vi "Actor Core.vi"(8 "error in":errorcluster, 11 "Nested in":refnum<class "GUI.lvclass">) -> (0 "error out":errorcluster, 3 "Actor out":refnum<class "Actor.lvclass">)   [LabVIEW 2020, in "GUI.lvlib" / "GUI.lvclass"]
doc: "(<B>Filename</B>: Actor Framework.lvlib:Actor.lvclass:Actor Core.vi)\n\nReceives messages to the actor, reacts to them, and initiates any error handling that may shut the actor down.\n\nDescendant classes may override this VI to append parallel tasks for the actor to complete while it handles messages. Overrides use the Call Parent Method node."
uses:
  GUI.lvclass
  C:/Program Files (x86)/National Instruments/LabVIEW 2020/vi.lib/ActorFramework/Actor/Actor.lvclass
  <vilib>/ActorFramework/Actor/Actor.lvclass
  <vilib>/ActorFramework/Message Enqueuer/Message Enqueuer.lvclass
  GUI.lvclass/GUI.ctl
  <vilib>/ActorFramework/Actor/Actor.lvclass/Actor.ctl
  <vilib>/ActorFramework/Message Enqueuer/Message Enqueuer.lvclass/Message Enqueuer.ctl
  <vilib>/ActorFramework/Stop Msg/Stop Msg.lvclass/Stop Msg.ctl
  Modbus/Modbus Messages/Control module to write Msg/Control module to write Msg.lvclass/Control module to write Msg.ctl
  <vilib>/ActorFramework/Message Enqueuer/Message Priority.ctl
  Modbus/Modbus Messages/Write to Module Msg/Write to Module Msg.lvclass/Write to Module Msg.ctl
  Modbus/Modbus/Modbus.lvclass
  Algorythm/Algorythm/Algorythm.lvclass
  <vilib>/ActorFramework/Message Enqueuer/Init from Existing Queue.vi
  <vilib>/ActorFramework/Message Enqueuer/Enqueue Critical.vi
  <vilib>/ActorFramework/Message Enqueuer/Enqueue.vi
  <vilib>/ActorFramework/Stop Msg/Stop Msg.lvclass
  C:/Program Files (x86)/National Instruments/LabVIEW 2020/vi.lib/ActorFramework/Message/Message.lvclass
  Modbus/Modbus Messages/Control module to write Msg/Control module to write Msg.lvclass
  Modbus/Modbus Messages/Write to Module Msg/Write to Module Msg.lvclass
  <vilib>/Utility/LVClass/Get LV Class Name.vi
  <resource>/AFDebug/Generate Trace for Message.vi
  <vilib>/ActorFramework/Message Priority Queue/Priority Enqueue.vi
  Setting Window.vi
panel:
  out "Alg end":bool
  out "Module Connect":bool
  out "LAI Connect":bool
  out "LDO Connect":bool
  out "LCP Connect":bool
  out "Modules States":u16
  in  "Serial num":string caption="S/n"
  in  "Stand_relays":T1
  in  "Settings":bool
  in  "Save Button":bool
  in  "Start Button":bool
  out "String Indicator":string
  out "Tab Control":enum32{"LAI", "LDO"}(tab)
  out "Control_lai_digi":T2
  out "Stand_lai":T3
  in  "Relays Control":T1
  out "Control_ldo":T3
  in  "Control Module":enum16{"LAI", "LDO"}(ring)
  out "Stand_lai_digi":T2
  in  "Connect":bool
  in  "Port":refnum<visa-resource-name> caption="Порт"
  out "Stand_lcp":T4
  out "Stand_lai":T3
  out "Stand_ldo":T3
  in  "Button 2":bool
  # "Стенд"
  # "Проверяемый модуль"
  # "Ход работы"
  # "LCP"
  # "LDO"
  # "LAI"
  # "LAI"
  # "LDO"
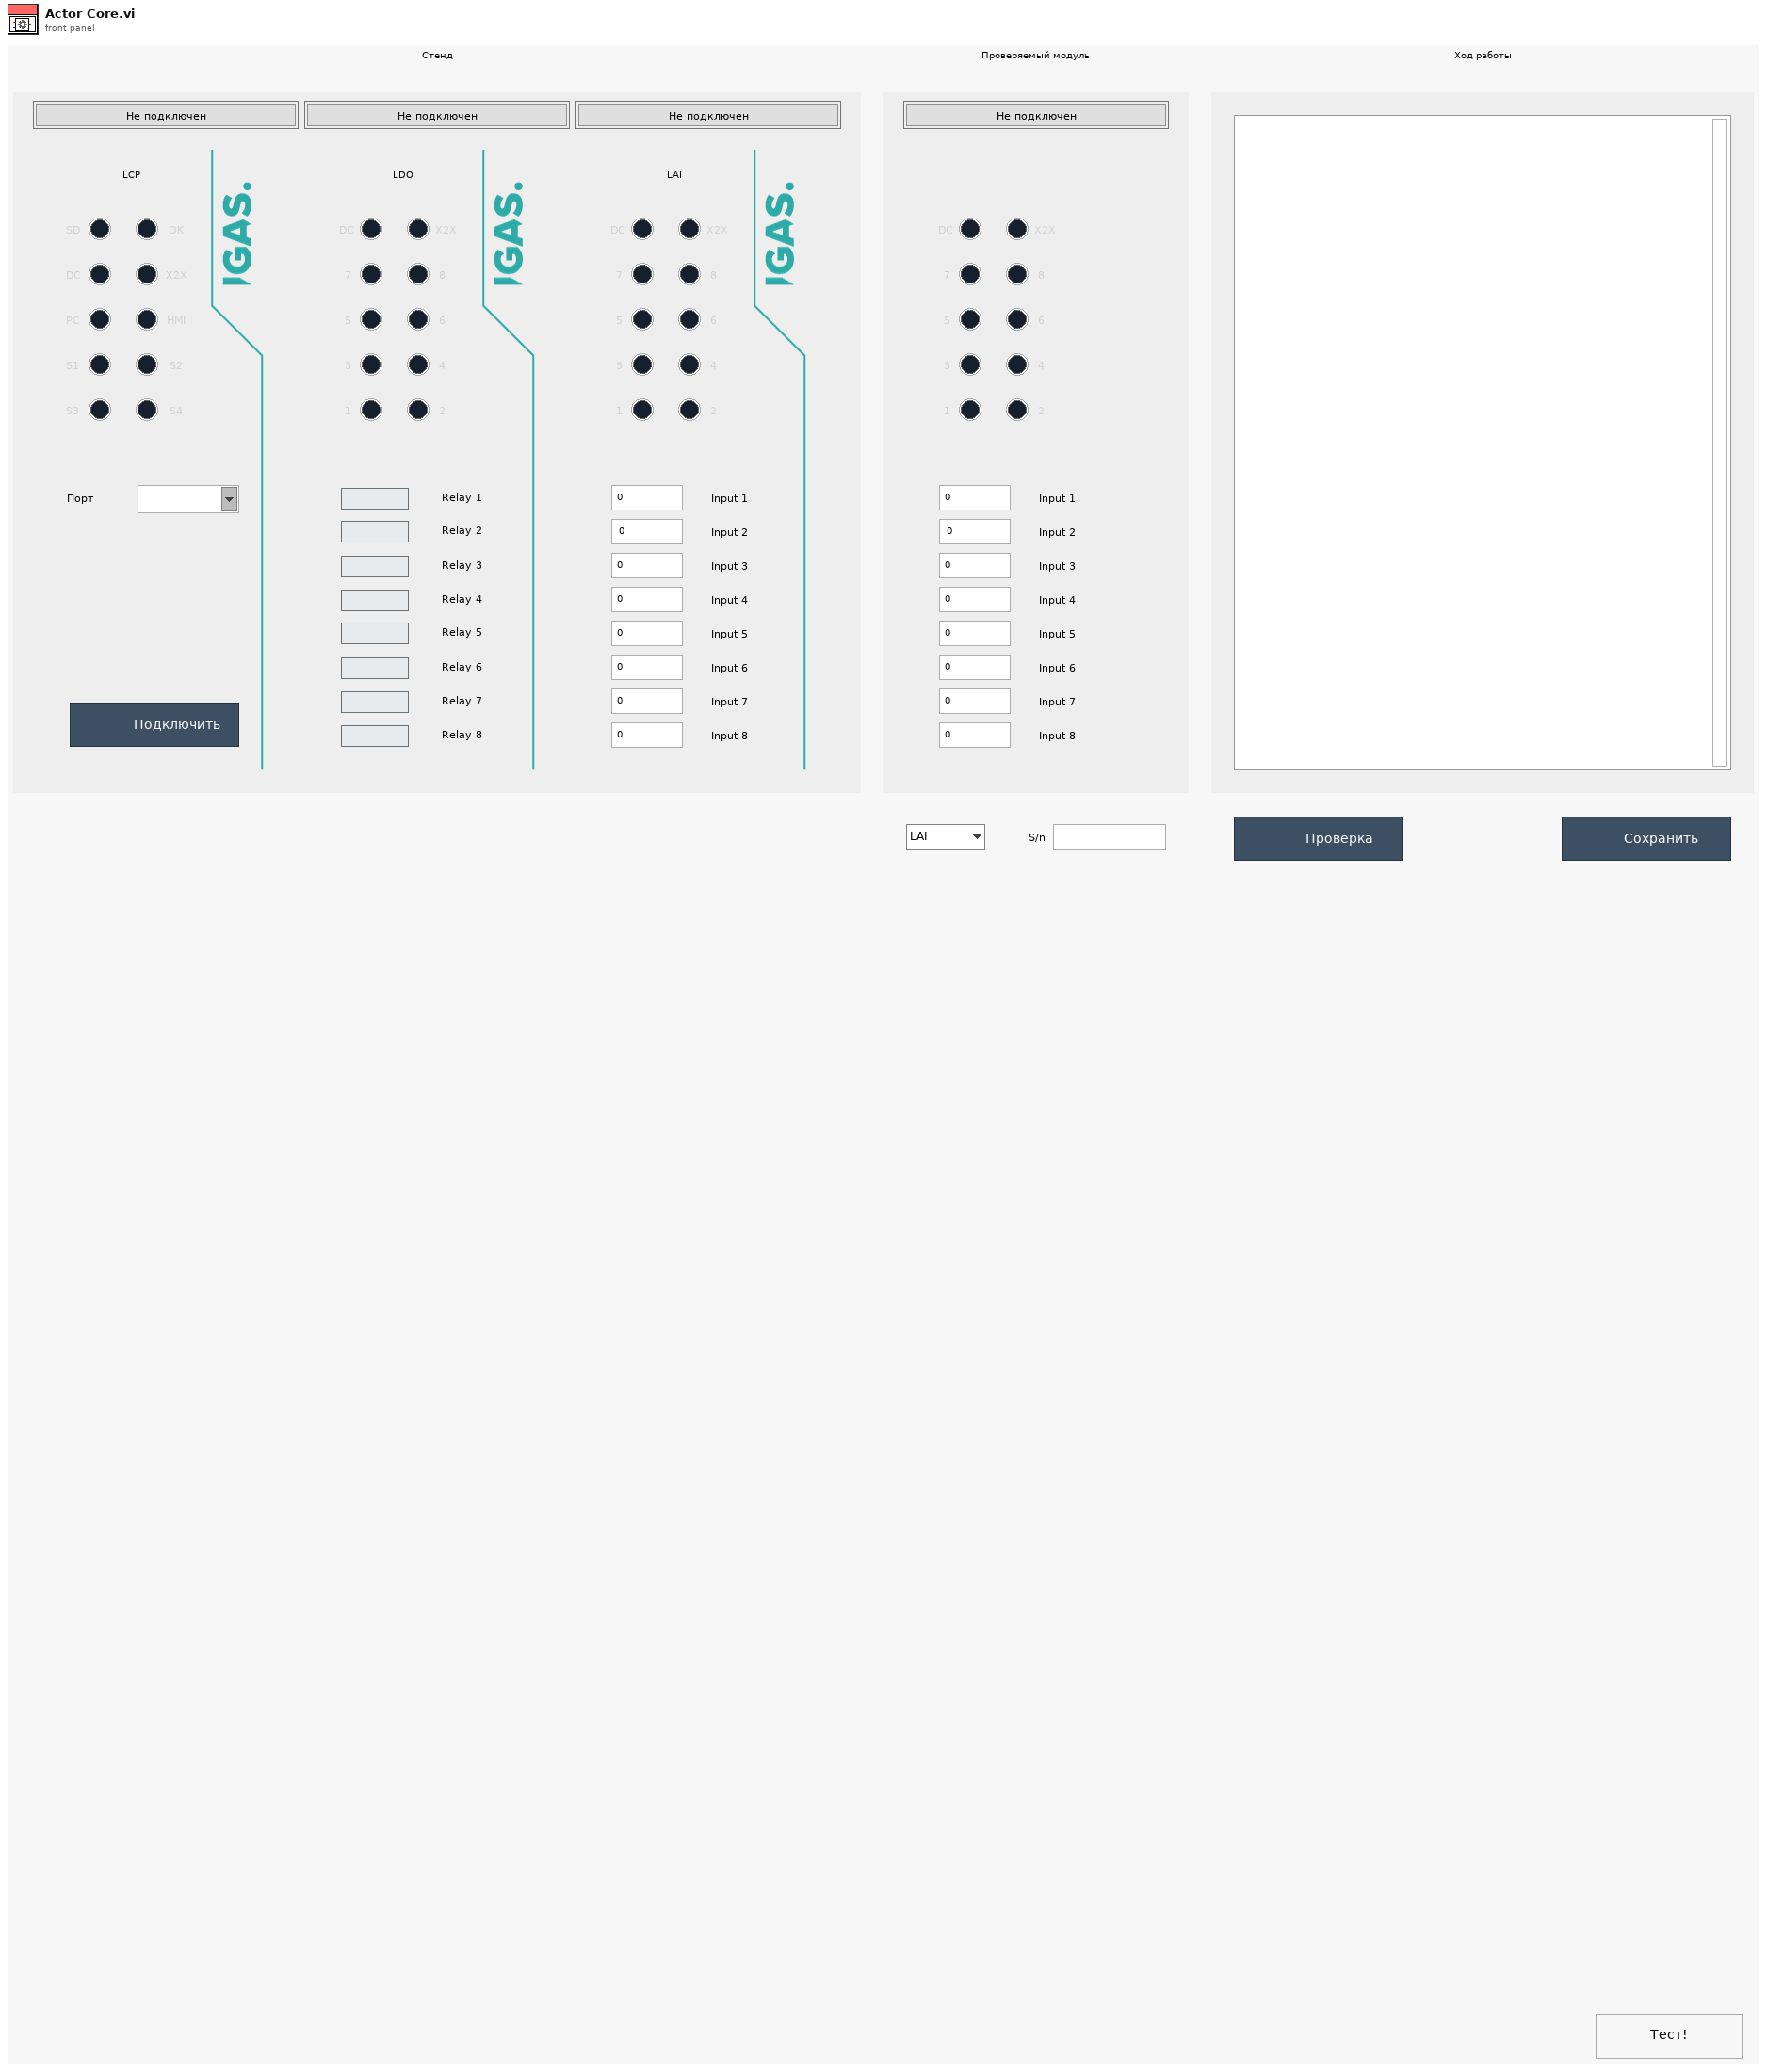
[diagram p1: front panel]
types:
  T1 = cluster{"Relay 1":bool, "Relay 2":bool, "Relay 3":bool, "Relay 4":bool, "Relay 5":bool, "Relay 6":bool, "Relay 7":bool, "Relay 8":bool}
  T2 = cluster{"Relay 16":dbl, "Relay 15":dbl, "Relay 14":dbl, "Relay 13":dbl, "Relay 12":dbl, "Relay 11":dbl, "Relay 10":dbl, "Relay 9":dbl}
  T3 = cluster{"Boolean 1":bool, "Boolean 2":bool, "Boolean 3":bool, "Boolean 4":bool, "Boolean 5":bool, "Boolean 6":bool, "Boolean 7":bool, "Boolean 8":bool, "Boolean 9":bool, "Boolean 10":bool}
  T4 = cluster{"Boolean 9":bool, "Boolean 7":bool, "Boolean 5":bool, "Boolean 3":bool, "Boolean 1":bool, "Boolean 10":bool, "Boolean 8":bool, "Boolean 6":bool, "Boolean 4":bool, "Boolean 2":bool}
  T5 = enum8{"Enabled", "Disabled", "Disabled and Grayed Out"}
  T6 = enum32{"Invalid", "Standard", "Closed", "Hidden", "Minimized", "Maximized"}
  T7 = cluster{"Stop":refnum<user-event>, "Stand_lcp":refnum<user-event>, "Stand_ldo":refnum<user-event>, "Stand_lai":refnum<user-event>, "Tab Control":refnum<user-event>, "Control_ldo":refnum<user-event>, "Modules States":refnum<user-event>, "Alg end":refnum<user-event>, "Update connection":refnum<user-event>}
  T8 = typedef "Port Settings.ctl" = cluster{"VISA resource":string, "BAUD":u16, "Parity":bool, "LDO":u16, "LAI":u16, "Control":u16, "Period":u16}
  T9 = typedef "Actor Framework.lvlib/Message Enqueuer.lvclass/Message Priority.ctl" = enum16{"Low", "Normal", "High"}
  T10 = enum16{"open", "replace", "create", "open or create", "replace or create", "replace or create with confirmation"}
  T11 = cluster{"[0]":dbl, "[1]":dbl, "[2]":dbl, "[3]":dbl, "[4]":dbl, "[5]":dbl, "[6]":dbl, "[7]":dbl}
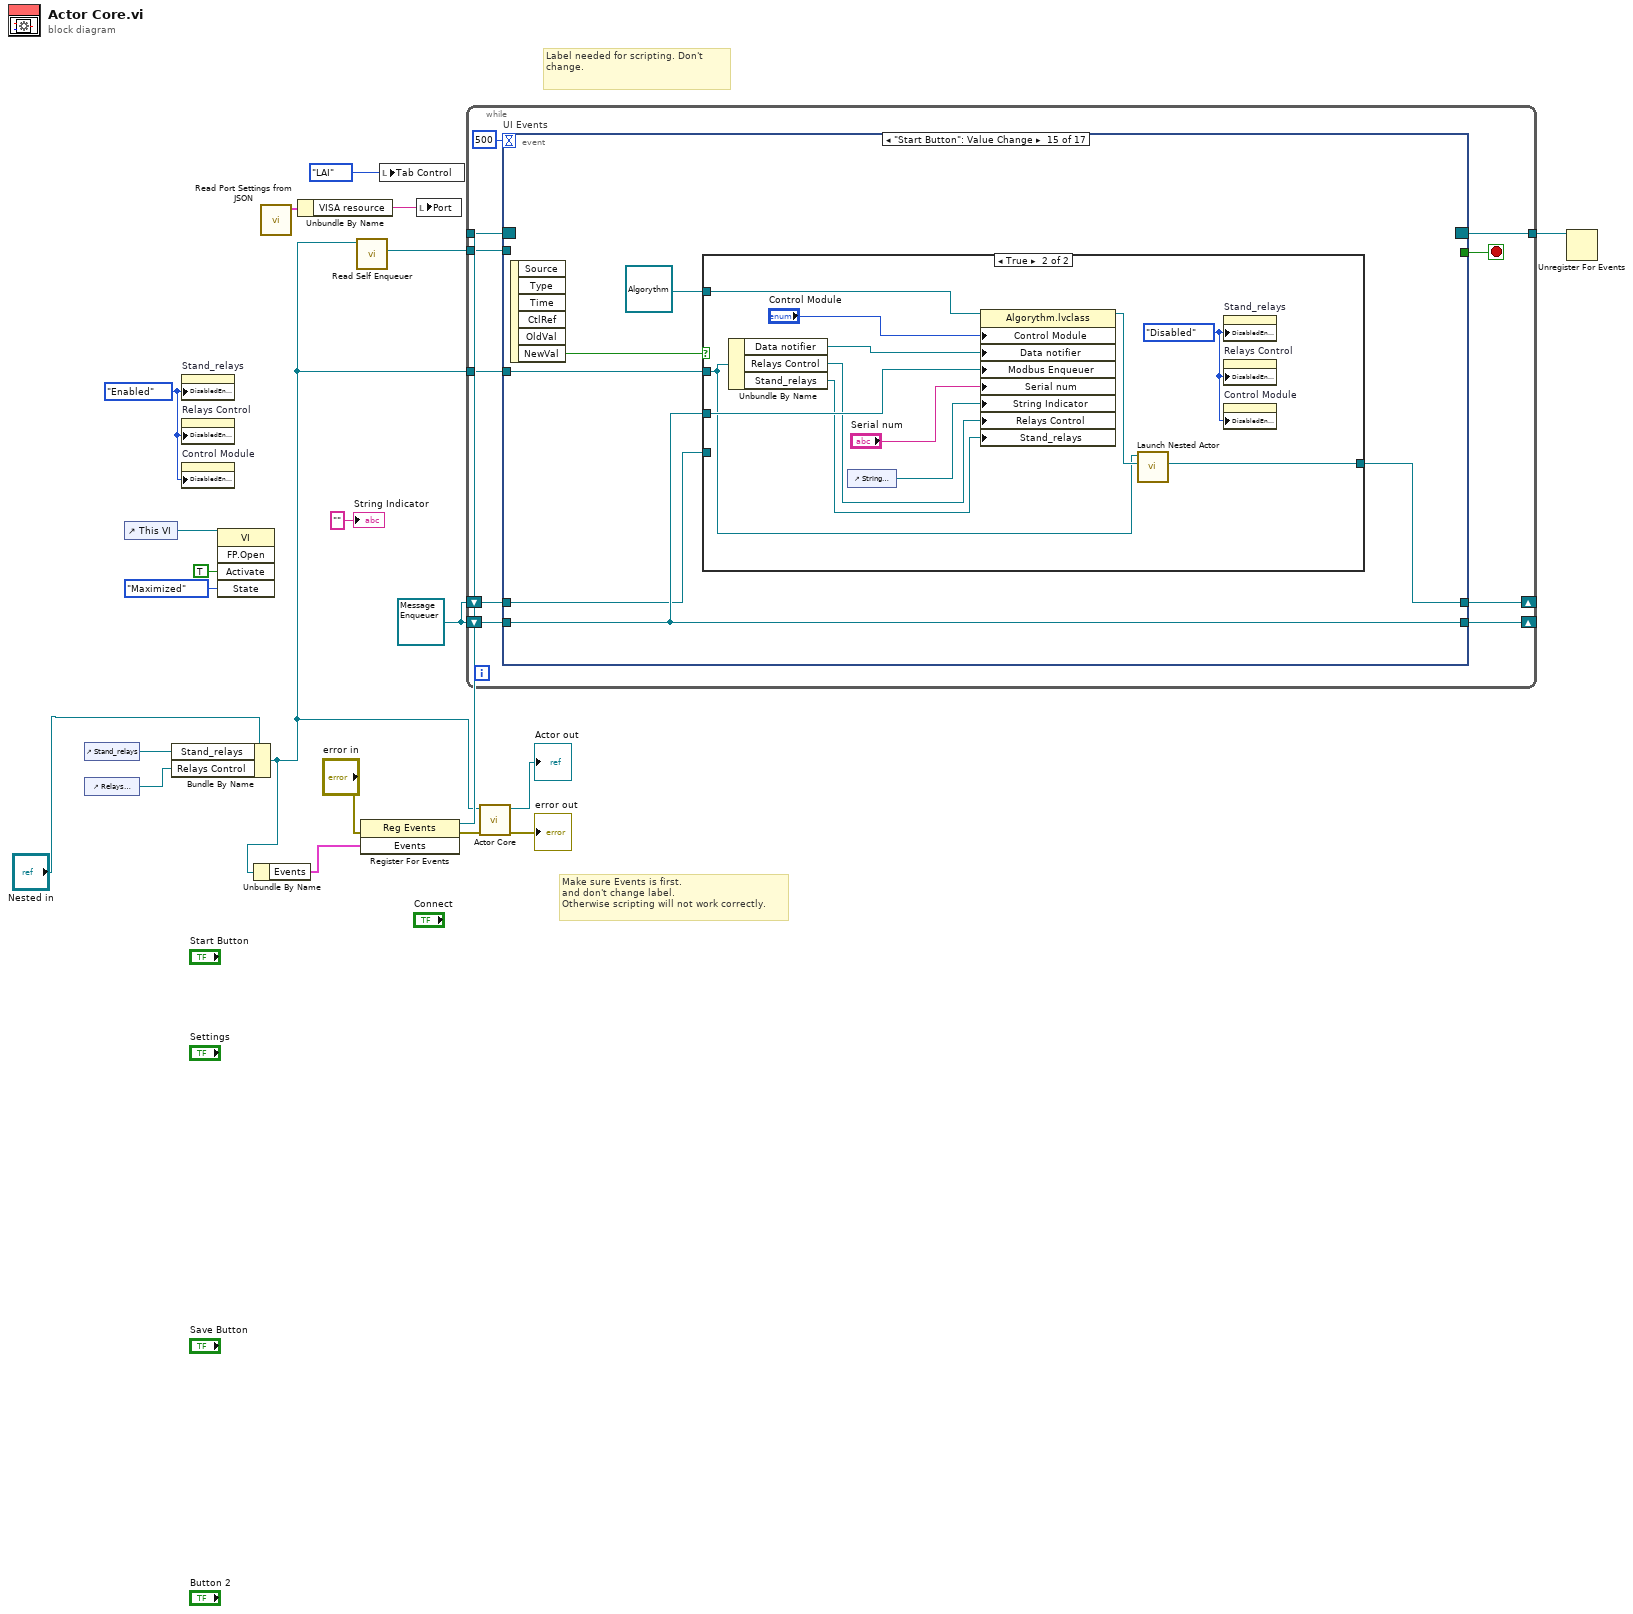
[diagram p0: block diagram]
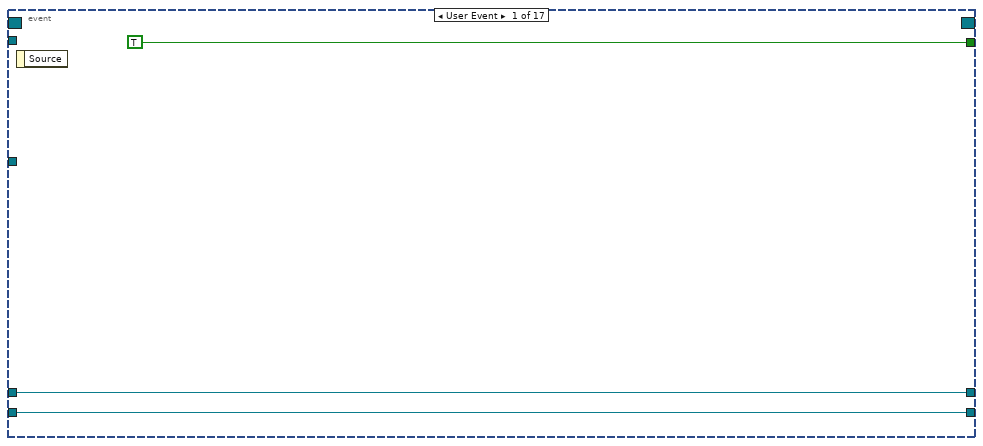
[diagram p2: hidden frame]
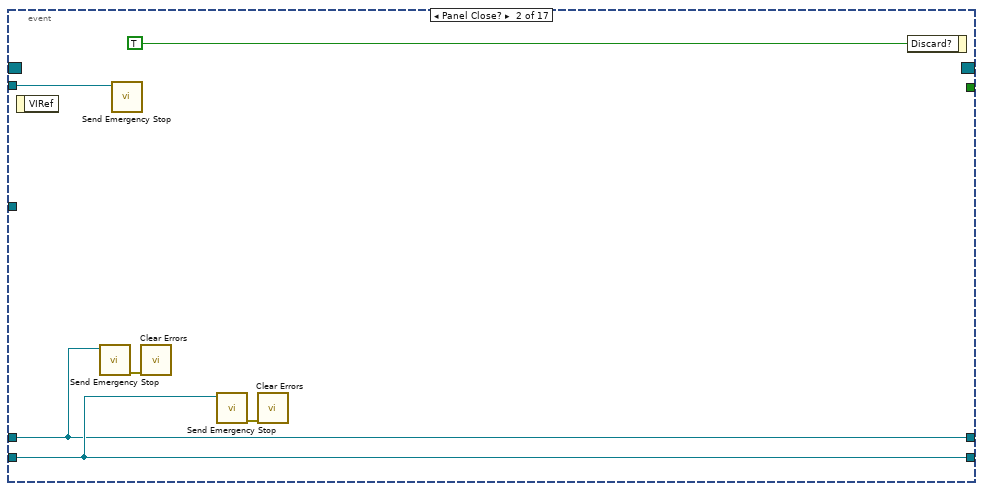
[diagram p3: hidden frame]
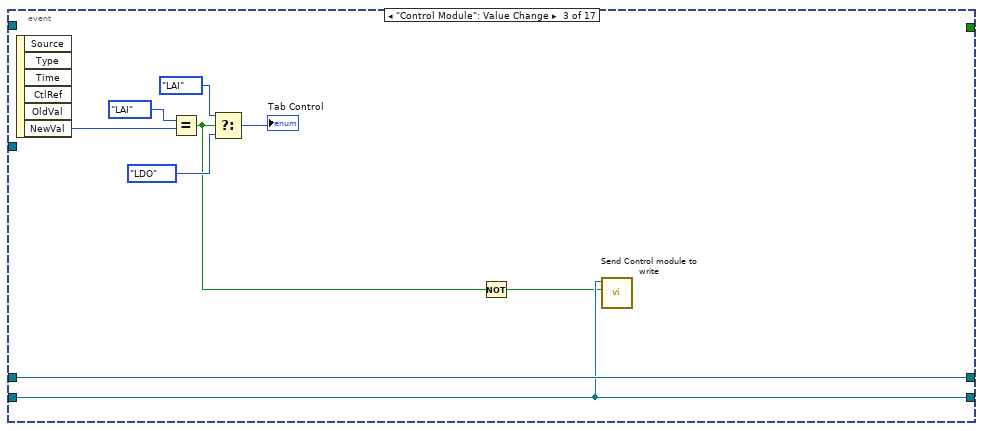
[diagram p4: hidden frame]
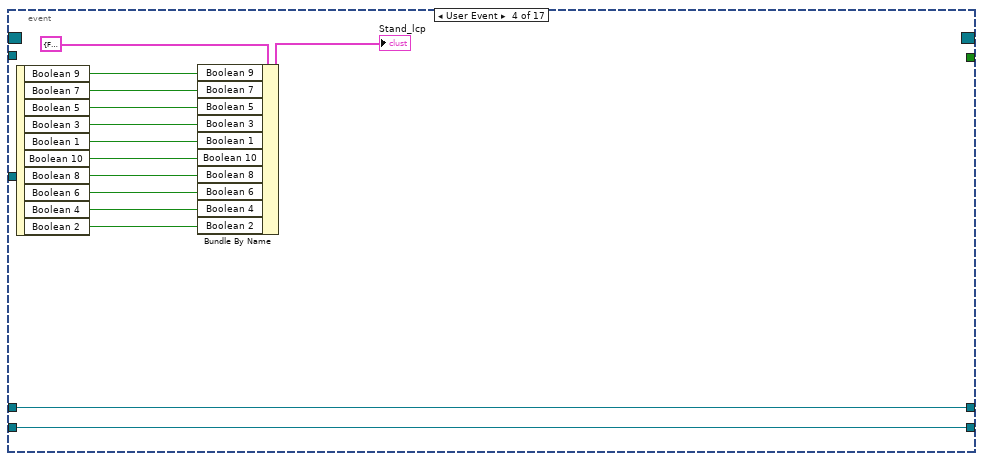
[diagram p5: hidden frame]
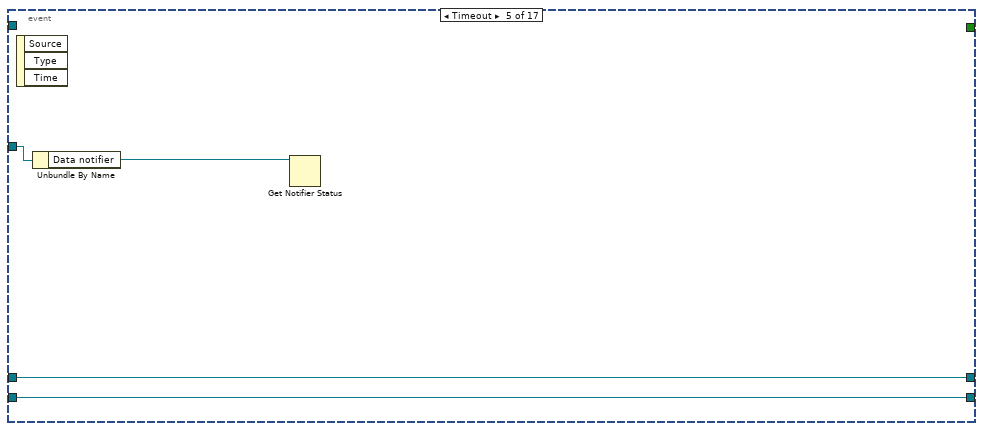
[diagram p6: hidden frame]
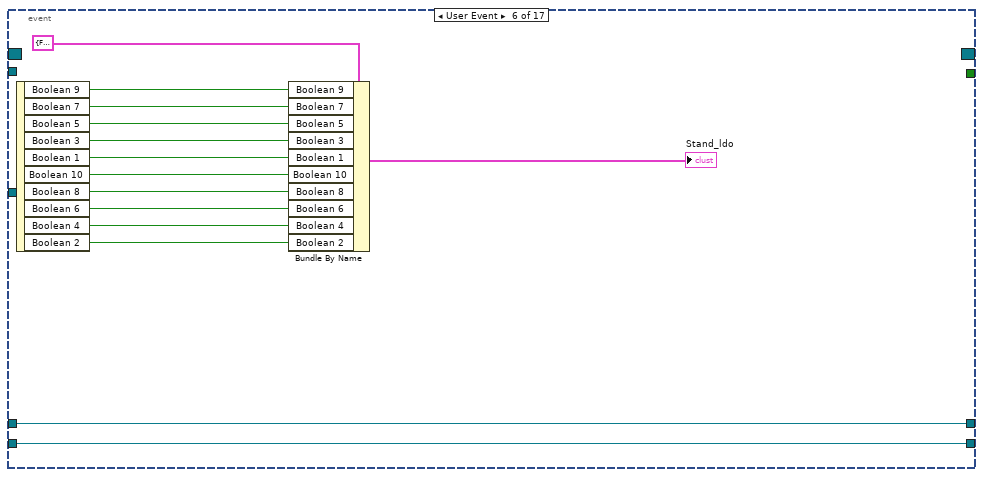
[diagram p7: hidden frame]
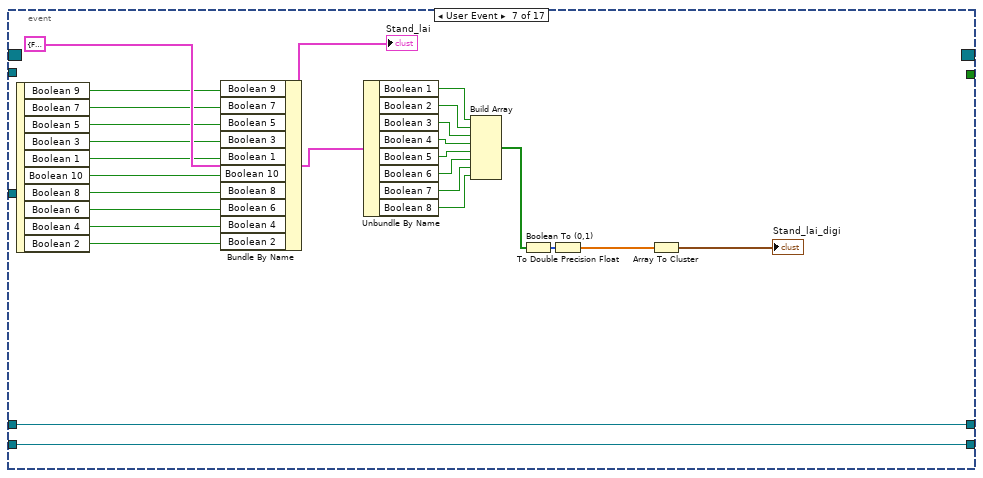
[diagram p8: hidden frame]
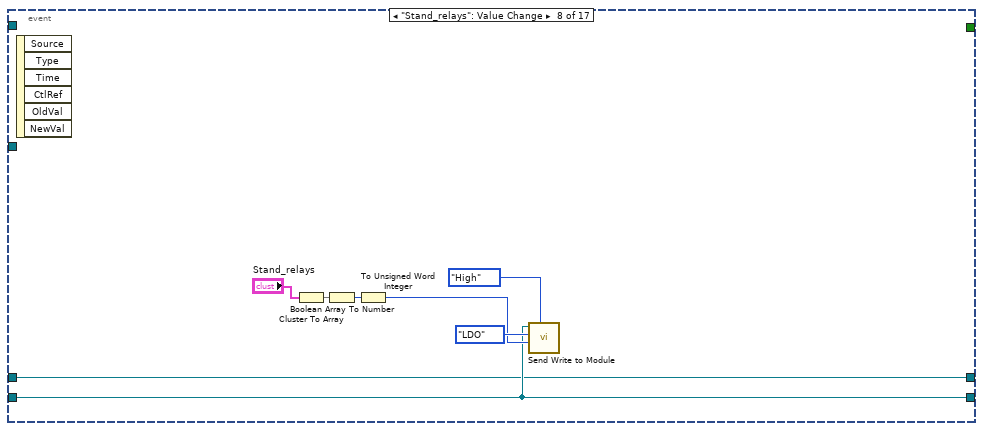
[diagram p9: hidden frame]
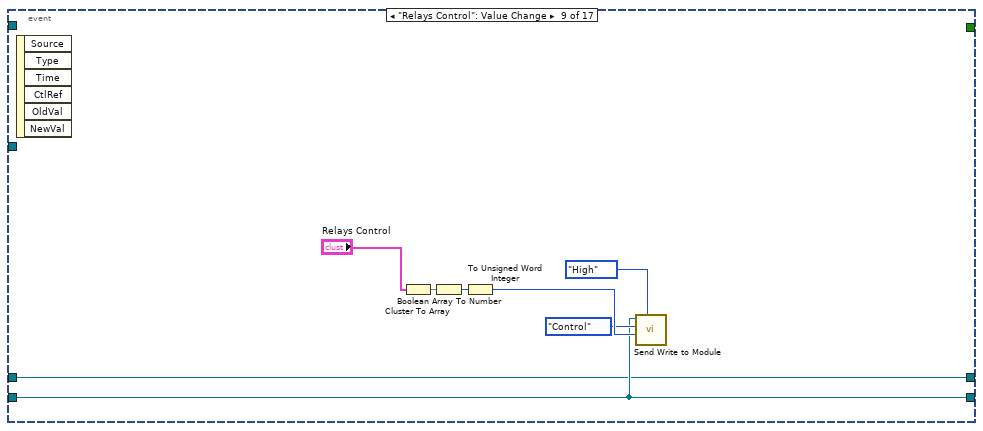
[diagram p10: hidden frame]
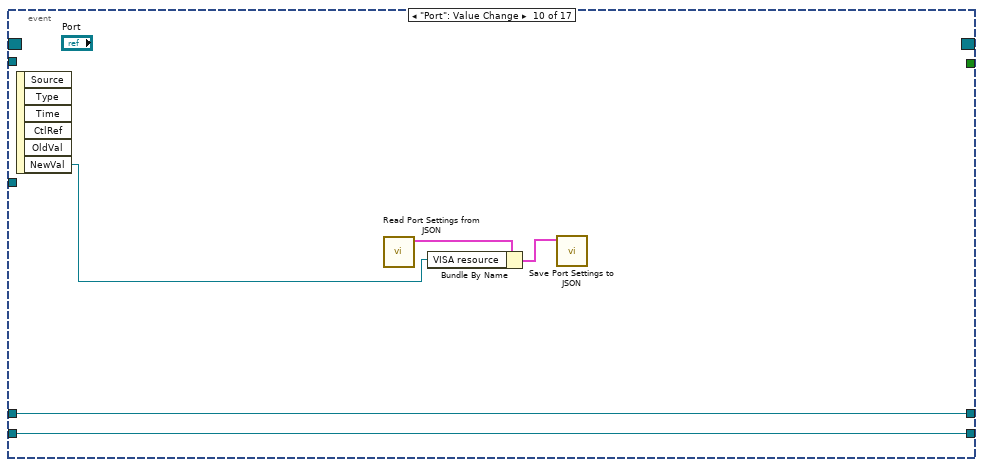
[diagram p11: hidden frame]
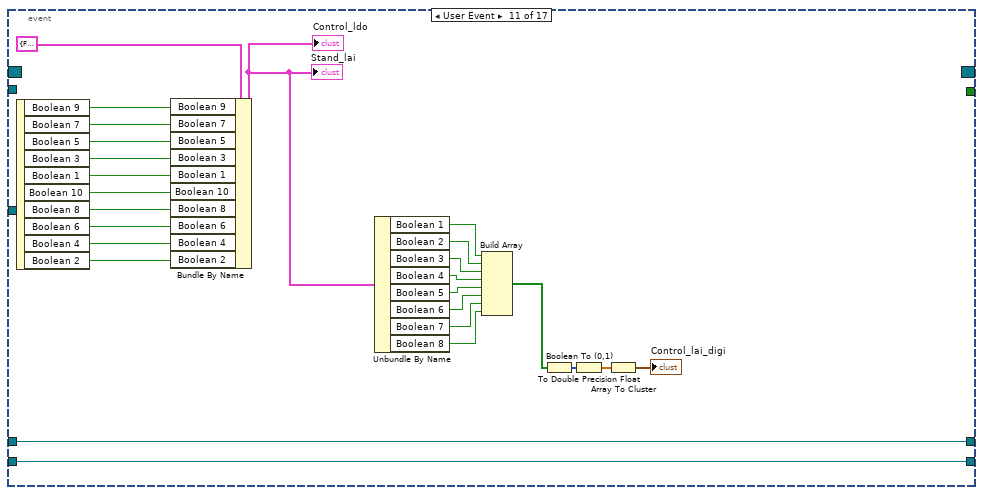
[diagram p12: hidden frame]
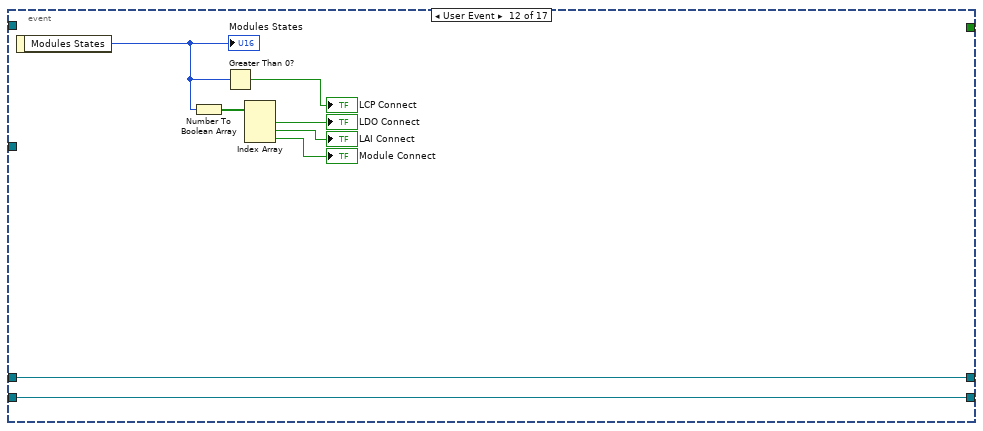
[diagram p13: hidden frame]
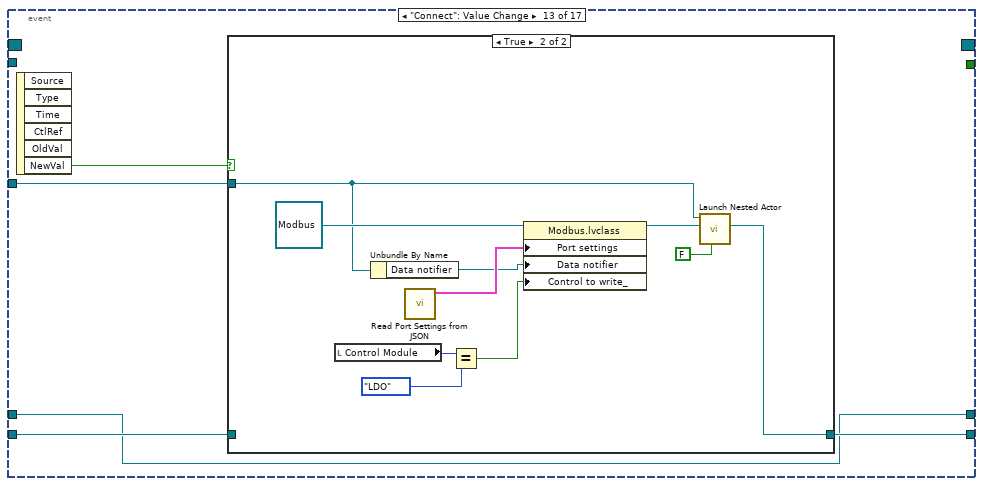
[diagram p14: hidden frame]
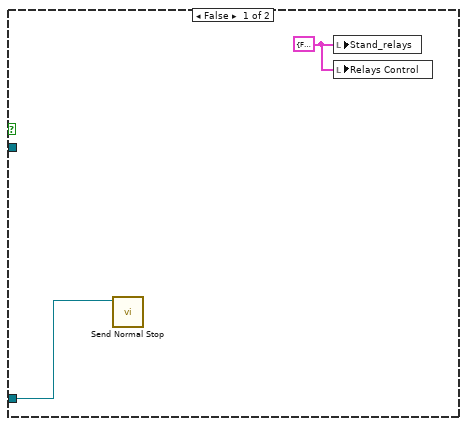
[diagram p15: hidden frame]
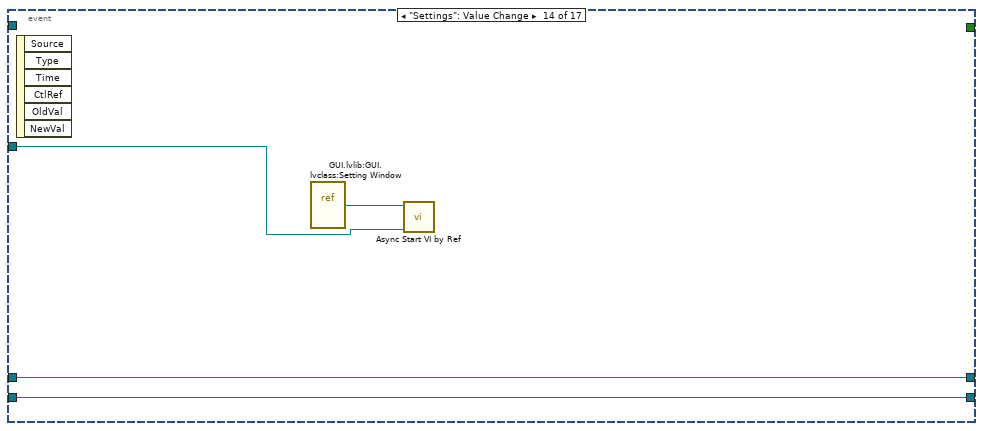
[diagram p16: hidden frame]
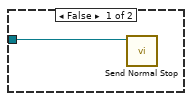
[diagram p17: hidden frame]
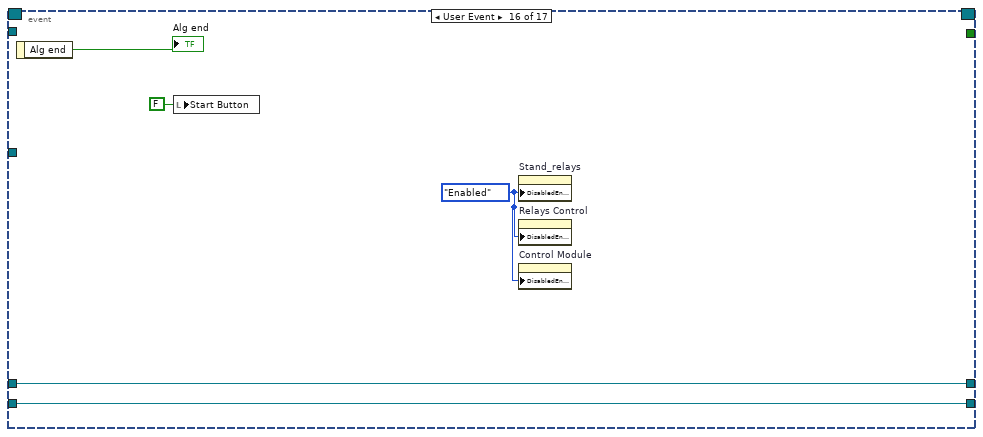
[diagram p18: hidden frame]
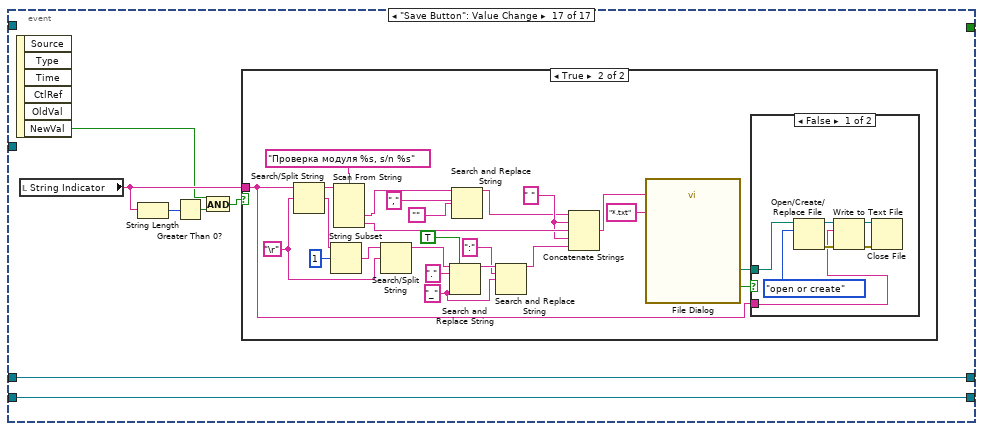
[diagram p19: hidden frame]
diagram:
  w1 = T5."Enabled" ("Disabled")
  w13 = refnum<class "Message Enqueuer.lvclass"> refnum ("Nested Actor's Enqueuer")
  # "Label needed for scripting. Don't change."
  # "Make sure Events is first.\nand don't change label.\nOtherwise scripting will not work correctly."
  n1 = control-ref of="Stand_relays"() -> (w11:refnum<vi>)
  n2 = control-ref of="Relays Control"() -> (w10:refnum<vi>)
  n3 = control-ref of="This VI"() -> (w7:refnum<vi>)
  n4 = Bundle By Name(cluster="Nested in", "Stand_relays"=w11, "Relays Control"=w10) -> (w9:refnum<class "GUI.lvclass">)
  n5 = property on="Stand_relays" class="Clust (strict)"("DisabledEnum"=w1) -> ()  [unwired: 2 in, 2 out]
  n6 = property on="Relays Control" class="Clust (strict)"("DisabledEnum"=w1) -> ()  [unwired: 2 in, 2 out]
  n7 = property on="Control Module" class="Enum (strict)"("DisabledEnum"=w1) -> ()  [unwired: 2 in, 2 out]
  n8 = invoke class="VI" method="FP.Open"(reference=w7, "Activate"=TRUE ("Activate?"), "State"=T6."Maximized") -> ()  [unwired: 2 in, 5 out]
  n9 = Unbundle By Name(w9) -> ("Events"=w18:T7)
  n10 = call "Read Port Settings from JSON.vi"() -> ("Port settings"=w4:T8)  [unwired: 11 in]
  n11 = Unbundle By Name(w4) -> ("VISA resource"=w3:string)
  n12 = call <vilib>:"Read Self Enqueuer.vi"("Actor"=w9) -> ("Self Enqueuer"=w16:refnum<class "Message Enqueuer.lvclass">)  [unwired: 10 in]
  n13 = register-events ("Main Register for Events")(error in="error in", w18) -> (reference out=w19:refnum<event-registration>, error out=w14:errorcluster)  [unwired: 1 in]
  n14 = local write "Tab Control"(enum32{"LAI", "LDO"}."LAI" ("Tab Control")) -> ()
  n15 = local write "Port"(w3) -> ()
  n16 = while {
    tunnel: w19 -> [w31]
    tunnel: [w29] -> w17
    tunnel: w16 -> [w28]
    tunnel: w9 -> [w27]
    shift-right: [w26] -> _
    shift-left: w13 -> [w25]
    shift-right: [w24] -> _
    shift-left: w13 -> [w23]
    stop <- w30 stop-if-true
    n17 = event "UI Events" shown="[14] \"Start Button\": Value Change" {
      selector: w31 -> [_ _ _ _ _ _ _ _ _ _ _ _ _ _ _ _ _]
      dyn-events: [_ _ _ _ _ _ _ _ _ _ _ _ _ _ _ _ _] -> w29
      timeout: 500 -> [_ _ _ _ _ _ _ _ _ _ _ _ _ _ _ _ _]
      tunnel: [TRUE _ _ _ _ _ _ _ _ _ _ _ _ _ _ _ _] -> w30
      tunnel: w28 -> [_ w39 _ _ _ _ _ _ _ _ _ _ _ _ _ _ _]
      tunnel: w27 -> [_ _ _ _ w65 _ _ _ _ _ _ _ w166 w180 w188 _ _]
      tunnel: [w33 w38 w43 w51 w67 w71 w96 w110 w119 w128 w143 w156 w165 w183 w187 w207 w214] -> w26
      tunnel: w25 -> [w33 w38 w43 w51 w67 w71 w96 w110 w119 w128 w143 w156 w164 w183 w187 w207 w214]
      tunnel: [w32 w35 w47 w50 w66 w70 w95 w109 w117 w127 w142 w155 w163 w182 w186 w206 w213] -> w24
      tunnel: w23 -> [w32 w35 w47 w50 w66 w70 w95 w109 w117 w127 w142 w155 w163 w182 w185 w206 w213]
      event User Event {
        n18 = event-data() -> ()  [unwired: 1 in, 1 out]
      }
      event Panel Close? {
        n19 = event-data() -> ()  [unwired: 1 in, 1 out]
        n20 = call <vilib>:"Send Emergency Stop.vi"("Message Enqueuer"=w35) -> ("error out"=w36:errorcluster)  [unwired: 10 in]
        n21 = call <vilib>:"Send Emergency Stop.vi"("Message Enqueuer"=w39) -> ()  [unwired: 10 in, 1 out]
        n22 = call <vilib>:"Clear Errors.vi"("error in (no error)"=w36) -> ()  [unwired: 5 in, 2 out]
        n23 = call <vilib>:"Send Emergency Stop.vi"("Message Enqueuer"=w38) -> ("error out"=w37:errorcluster)  [unwired: 10 in]
        n24 = call <vilib>:"Clear Errors.vi"("error in (no error)"=w37) -> ()  [unwired: 5 in, 2 out]
        n25 = event-data("Discard?"=TRUE) -> ()  [unwired: 1 in, 1 out]
      }
      event "Control Module": Value Change {
        n26 = event-data() -> ("NewVal"=w49:enum16{"LAI", "LDO"})  [unwired: 1 in, 5 out]
        n27 = Equal?(x=enum16{"LAI", "LDO"}."LAI", y=w49) -> (x = y?=w41:bool)
        n28 = Select(t=enum32{"LAI", "LDO"}."LAI" ("Tab Control"), s=w41, f=enum32{"LAI", "LDO"}."LDO" ("Tab Control")) -> (s? t:f=→"Tab Control":enum32{"LAI", "LDO"})
        n29 = Not(x=w41) -> (.not. x?=w42:bool)
        n30 = call "Send Control module to write.vi"("Control to write?"=w42, "Message Enqueuer"=w43) -> ()  [unwired: 8 in, 2 out]
      }
      event User Event {
        n31 = event-data() -> ("Boolean 9"=w62:bool, "Boolean 7"=w61:bool, "Boolean 5"=w60:bool, "Boolean 3"=w59:bool, "Boolean 1"=w58:bool, "Boolean 10"=w57:bool, "Boolean 8"=w56:bool, "Boolean 6"=w55:bool, "Boolean 4"=w54:bool, "Boolean 2"=w53:bool)  [unwired: 1 in]
        n32 = Bundle By Name(cluster=T4 {"Boolean 9"=FALSE, "Boolean 7"=FALSE, "Boolean 5"=FALSE, "Boolean 3"=FALSE, "Boolean 1"=FALSE, "Boolean 10"=FALSE, "Boolean 8"=FALSE, "Boolean 6"=FALSE, "Boolean 4"=FALSE, "Boolean 2"=FALSE} ("Stand_lcp"), "Boolean 9"=w62, "Boolean 7"=w61, "Boolean 5"=w60, "Boolean 3"=w59, "Boolean 1"=w58, "Boolean 10"=w57, "Boolean 8"=w56, "Boolean 6"=w55, "Boolean 4"=w54, "Boolean 2"=w53) -> (→"Stand_lcp":T4)
      }
      event Timeout {
        n33 = event-data() -> ()  [unwired: 1 in, 3 out]
        n34 = Unbundle By Name(w65) -> ("Data notifier"=w64:refnum<notifier>)
        n35 = Get Notifier Status(notifier=w64) -> ()  [unwired: 1 in, 5 out]
      }
      event User Event {
        n36 = event-data() -> ("Boolean 9"=w81:bool, "Boolean 7"=w80:bool, "Boolean 5"=w79:bool, "Boolean 3"=w78:bool, "Boolean 1"=w77:bool, "Boolean 10"=w76:bool, "Boolean 8"=w75:bool, "Boolean 6"=w74:bool, "Boolean 4"=w73:bool, "Boolean 2"=w72:bool)  [unwired: 1 in]
        n37 = Bundle By Name(cluster=T4 {"Boolean 9"=FALSE, "Boolean 7"=FALSE, "Boolean 5"=FALSE, "Boolean 3"=FALSE, "Boolean 1"=FALSE, "Boolean 10"=FALSE, "Boolean 8"=FALSE, "Boolean 6"=FALSE, "Boolean 4"=FALSE, "Boolean 2"=FALSE} ("Stand_ldo"), "Boolean 9"=w81, "Boolean 7"=w80, "Boolean 5"=w79, "Boolean 3"=w78, "Boolean 1"=w77, "Boolean 10"=w76, "Boolean 8"=w75, "Boolean 6"=w74, "Boolean 4"=w73, "Boolean 2"=w72) -> (→"Stand_ldo":T4)
      }
      event User Event {
        n38 = event-data() -> ("Boolean 9"=w106:bool, "Boolean 7"=w105:bool, "Boolean 5"=w104:bool, "Boolean 3"=w103:bool, "Boolean 1"=w102:bool, "Boolean 10"=w101:bool, "Boolean 8"=w100:bool, "Boolean 6"=w99:bool, "Boolean 4"=w98:bool, "Boolean 2"=w97:bool)  [unwired: 1 in]
        n39 = Bundle By Name(cluster=T4 {"Boolean 9"=FALSE, "Boolean 7"=FALSE, "Boolean 5"=FALSE, "Boolean 3"=FALSE, "Boolean 1"=FALSE, "Boolean 10"=FALSE, "Boolean 8"=FALSE, "Boolean 6"=FALSE, "Boolean 4"=FALSE, "Boolean 2"=FALSE} ("Stand_lai"), "Boolean 9"=w106, "Boolean 7"=w105, "Boolean 5"=w104, "Boolean 3"=w103, "Boolean 1"=w102, "Boolean 10"=w101, "Boolean 8"=w100, "Boolean 6"=w99, "Boolean 4"=w98, "Boolean 2"=w97) -> (w91:T4)
        "Stand_lai" <- w91
        n40 = Unbundle By Name(w91) -> ("Boolean 1"=w90:bool, "Boolean 2"=w88:bool, "Boolean 3"=w87:bool, "Boolean 4"=w89:bool, "Boolean 5"=w86:bool, "Boolean 6"=w83:bool, "Boolean 7"=w84:bool, "Boolean 8"=w85:bool)
        n41 = Build Array(w90, w88, w87, w89, w86, w83, w84, w85) -> (w82:bool[])
        n42 = Boolean To (0,1)(Boolean=w82) -> (0, 1=w93:i16[])
        n43 = To Double Precision Float(number=w93) -> (double precision float=w92:dbl[])
        n44 = Array To Cluster(array=w92) -> (cluster=→"Stand_lai_digi":T11)
      }
      event "Stand_relays": Value Change {
        n45 = event-data() -> ()  [unwired: 1 in, 6 out]
        n46 = Cluster To Array(cluster="Stand_relays") -> (array=w113:bool[])
        n47 = Boolean Array To Number(Boolean array=w113) -> (number=w112:u32)
        n48 = To Unsigned Word Integer(number=w112) -> (unsigned 16bit integer=w111:u16)
        n49 = call "Send Write to Module.vi"("Message Priority (Normal)"=Message_Priority."High", "Data"=w111, "Module"=enum16{"LAI", "LDO", "Control"}."LDO", "Message Enqueuer"=w110) -> ()  [unwired: 6 in, 2 out]
      }
      event "Relays Control": Value Change {
        n50 = event-data() -> ()  [unwired: 1 in, 6 out]
        n51 = Cluster To Array(cluster="Relays Control") -> (array=w123:bool[])
        n52 = Boolean Array To Number(Boolean array=w123) -> (number=w122:u32)
        n53 = To Unsigned Word Integer(number=w122) -> (unsigned 16bit integer=w121:u16)
        n54 = call "Send Write to Module.vi"("Message Priority (Normal)"=Message_Priority."High", "Data"=w121, "Module"=enum16{"LAI", "LDO", "Control"}."Control", "Message Enqueuer"=w119) -> ()  [unwired: 6 in, 2 out]
      }
      event "Port": Value Change {
        n55 = event-data() -> ("NewVal"=w124:refnum<visa-resource-name>)  [unwired: 1 in, 5 out]
        n56 = call "Read Port Settings from JSON.vi"() -> ("Port settings"=w126:T8)  [unwired: 11 in]
        n57 = Bundle By Name(cluster=w126, "VISA resource"=w124) -> (w125:T8)
        n58 = call "Save Port Settings to JSON.vi"("Port settings"=w125) -> ()  [unwired: 11 in]
      }
      event User Event {
        n59 = event-data() -> ("Boolean 9"=w153:bool, "Boolean 7"=w152:bool, "Boolean 5"=w151:bool, "Boolean 3"=w150:bool, "Boolean 1"=w149:bool, "Boolean 10"=w148:bool, "Boolean 8"=w147:bool, "Boolean 6"=w146:bool, "Boolean 4"=w145:bool, "Boolean 2"=w144:bool)  [unwired: 1 in]
        n60 = Bundle By Name(cluster=T4 {"Boolean 9"=FALSE, "Boolean 7"=FALSE, "Boolean 5"=FALSE, "Boolean 3"=FALSE, "Boolean 1"=FALSE, "Boolean 10"=FALSE, "Boolean 8"=FALSE, "Boolean 6"=FALSE, "Boolean 4"=FALSE, "Boolean 2"=FALSE} ("Control_ldo"), "Boolean 9"=w153, "Boolean 7"=w152, "Boolean 5"=w151, "Boolean 3"=w150, "Boolean 1"=w149, "Boolean 10"=w148, "Boolean 8"=w147, "Boolean 6"=w146, "Boolean 4"=w145, "Boolean 2"=w144) -> (w130:T4)
        "Control_ldo" <- w130
        "Stand_lai" <- w130
        n61 = Unbundle By Name(w130) -> ("Boolean 1"=w138:bool, "Boolean 2"=w136:bool, "Boolean 3"=w135:bool, "Boolean 4"=w137:bool, "Boolean 5"=w134:bool, "Boolean 6"=w131:bool, "Boolean 7"=w132:bool, "Boolean 8"=w133:bool)
        n62 = Build Array(w138, w136, w135, w137, w134, w131, w132, w133) -> (w129:bool[])
        n63 = Boolean To (0,1)(Boolean=w129) -> (0, 1=w141:i16[])
        n64 = To Double Precision Float(number=w141) -> (double precision float=w140:dbl[])
        n65 = Array To Cluster(array=w140) -> (cluster=→"Control_lai_digi":T11)
      }
      event User Event {
        n66 = event-data() -> ("Modules States"=w158:u16)  [unwired: 1 in]
        "Modules States" <- w158
        n67 = Number To Boolean Array(number=w158) -> (Boolean array=w162:bool[])
        n68 = Greater Than 0?(x=w158) -> (x > 0?=→"LCP Connect":bool)
        n69 = Index Array(array=w162) -> (element #1=→"LDO Connect":bool, element #2=→"LAI Connect":bool, element #3=→"Module Connect":bool)  [unwired: 3 in]
      }
      event "Connect": Value Change {
        n70 = event-data() -> ("NewVal"=w167:bool)  [unwired: 1 in, 5 out]
        n71 = case shown="True" w167 {
          tunnel: w166 -> [_ w174]
          tunnel: [_ w177] -> w165
          tunnel: w164 -> [w169 _]
          frame False {
            w168 = T1 {"Relay 1"=FALSE, "Relay 2"=FALSE, "Relay 3"=FALSE, "Relay 4"=FALSE, "Relay 5"=FALSE, "Relay 6"=FALSE, "Relay 7"=FALSE, "Relay 8"=FALSE} ("Stand_relays")
            n72 = call <vilib>:"Send Normal Stop.vi"("Message Enqueuer"=w169) -> ()  [unwired: 10 in, 1 out]
            n73 = local write "Stand_relays"(w168) -> ()
            n74 = local write "Relays Control"(w168) -> ()
          }
          frame True {
            n75 = local read "Control Module"() -> (w172:enum16{"LAI", "LDO"})
            n76 = Unbundle By Name(w174) -> ("Data notifier"=w173:refnum<notifier>)
            n77 = call "Read Port Settings from JSON.vi"() -> ("Port settings"=w175:T8)  [unwired: 11 in]
            n78 = Equal?(x=w172, y=enum16{"LAI", "LDO"}."LDO") -> (x = y?=w170:bool)
            n79 = property class="Modbus.lvclass"(reference=refnum<class "Modbus.lvclass"> refnum ("Modbus.lvlib:Modbus.lvclass"), "Port settings"=w175, "Data notifier"=w173, "Control to write_"=w170) -> (reference out=w178:refnum<class "Modbus.lvclass">)  [unwired: 1 in, 1 out]
            n80 = call <vilib>:"Launch Nested Actor.vi"("Open Actor Core front panel? (F)"=FALSE, "Nested Actor"=w178, "Caller Actor in"=w174) -> ("Nested Actor's Enqueuer"=w177:refnum<class "Message Enqueuer.lvclass">)  [unwired: 6 in, 2 out]
          }
        }
      }
      event "Settings": Value Change {
        n81 = event-data() -> ()  [unwired: 1 in, 6 out]
        n82 = vi-ref "GUI.lvlib:GUI.lvclass:Setting Window.vi"() -> (w181:refnum<vi>)
        n83 = call "Async Start VI by Ref.vi"("GUI.lvlib:GUI.lvclass"=w180, "Static VI reference"=w181) -> ()  [unwired: 10 in]
      }
      event "Start Button": Value Change {
        n84 = event-data() -> ("NewVal"=w189:bool)  [unwired: 1 in, 5 out]
        n85 = case shown="True" w189 {
          tunnel: w188 -> [_ w196]
          tunnel: w187 -> [_ w200]
          tunnel: w185 -> [w190 _]
          tunnel: [_ w195] -> w186
          tunnel: refnum<class "Algorythm.lvclass"> refnum ("Algorythm.lvlib:Algorythm.lvclass") -> [_ w192]
          frame False {
            n86 = call <vilib>:"Send Normal Stop.vi"("Message Enqueuer"=w190) -> ()  [unwired: 10 in, 1 out]
          }
          frame True {
            w191 = T5."Disabled" ("Disabled")
            n87 = Unbundle By Name(w196) -> ("Data notifier"=w201:refnum<notifier>, "Relays Control"=w194:refnum<vi>, "Stand_relays"=w193:refnum<vi>)
            n88 = control-ref of="String Indicator"() -> (w198:refnum<vi>)
            n89 = property class="Algorythm.lvclass"(reference=w192, "Control Module"="Control Module", "Data notifier"=w201, "Modbus Enqueuer"=w200, "Serial num"="Serial num", "String Indicator"=w198, "Relays Control"=w194, "Stand_relays"=w193) -> (reference out=w197:refnum<class "Algorythm.lvclass">)  [unwired: 1 in, 1 out]
            n90 = call <vilib>:"Launch Nested Actor.vi"("Nested Actor"=w197, "Caller Actor in"=w196) -> ("Nested Actor's Enqueuer"=w195:refnum<class "Message Enqueuer.lvclass">)  [unwired: 7 in, 2 out]
            n91 = property on="Stand_relays" class="Clust (strict)"("DisabledEnum"=w191) -> ()  [unwired: 2 in, 2 out]
            n92 = property on="Relays Control" class="Clust (strict)"("DisabledEnum"=w191) -> ()  [unwired: 2 in, 2 out]
            n93 = property on="Control Module" class="Enum (strict)"("DisabledEnum"=w191) -> ()  [unwired: 2 in, 2 out]
          }
        }
      }
      event User Event {
        w203 = T5."Enabled" ("Disabled")
        n94 = event-data() -> ("Alg end"=→"Alg end":bool)  [unwired: 1 in]
        n95 = local write "Start Button"(FALSE ("Start Button")) -> ()
        n96 = property on="Stand_relays" class="Clust (strict)"("DisabledEnum"=w203) -> ()  [unwired: 2 in, 2 out]
        n97 = property on="Relays Control" class="Clust (strict)"("DisabledEnum"=w203) -> ()  [unwired: 2 in, 2 out]
        n98 = property on="Control Module" class="Enum (strict)"("DisabledEnum"=w203) -> ()  [unwired: 2 in, 2 out]
      }
      event "Save Button": Value Change {
        n99 = event-data() -> ("NewVal"=w208:bool)  [unwired: 1 in, 5 out]
        n100 = local read "String Indicator"() -> (w212:string)
        n101 = String Length(string=w212) -> (length=w211:i32)
        n102 = Greater Than 0?(x=w211) -> (x > 0?=w210:bool)
        n103 = And(x=w208, y=w210) -> (x .and. y?=w209:bool)
        n104 = case shown="True" w209 {
          tunnel: w212 -> [_ w220]
          frame False {
          }
          frame True {
            w225 = " " ("string")
            w227 = "_" ("replace string (\"\")")
            w233 = "\r"
            n105 = Search/Split String(string=w220, search string/char (-)=w233) -> (substring before match=w237:string, match + rest of string=w236:string)  [unwired: 1 in, 1 out]
            n106 = String Subset(string=w236, offset (0)=1) -> (substring=w234:string)  [unwired: 1 in]
            n107 = Scan From String(format string="Проверка модуля %s, s/n %s", input string=w237) -> (output 1=w218:string, output 2=w226:string)  [unwired: 4 in, 3 out]
            n108 = Search/Split String(string=w234, search string/char (-)=w233) -> (substring before match=w231:string)  [unwired: 1 in, 2 out]
            n109 = Search and Replace String(replace all?=TRUE ("replace all? (F)"), input string=w231, search string=".", replace string=w227) -> (result string=w229:string)  [unwired: 4 in, 3 out]
            n110 = Search and Replace String(input string=w218, search string=",", replace string="") -> (result string=w215:string)  [unwired: 5 in, 3 out]
            n111 = Search and Replace String(input string=w229, search string=":", replace string=w227) -> (result string=w224:string)  [unwired: 5 in, 3 out]
            n112 = Concatenate Strings(w215, w225, w226, w225, w224) -> (w219:string)
            n113 = call "File Dialog"("default name"=w219, "pattern (all files)"="*.txt") -> ("selected path"=w221:path, "cancelled"=w222:bool)  [unwired: 10 in, 2 out]
            n114 = case shown="False" w222 {
              tunnel: w221 -> [w245 _]
              tunnel: w220 -> [w241 _]
              frame False {
                n115 = Open/Create/Replace File(file path (use dialog)=w245, operation (0:open)=T10."open or create") -> (refnum out=w242:refnum<file>, error out=w243:errorcluster)  [unwired: 4 in, 1 out]
                n116 = Write to Text File(file (use dialog)=w242, text=w241, error in=w243) -> (refnum out=w239:refnum<file>, error out=w240:errorcluster)  [unwired: 1 in, 1 out]
                n117 = Close File(refnum=w239, error in=w240) -> ()  [unwired: 2 out]
              }
              frame True {
              }
            }
          }
        }
      }
    }
  }
  n118 = call-parent "Actor Core.vi"("error in"=w14, "Actor in"=w9) -> ("error out"=→"error out":errorcluster, "Actor out"=→"Actor out":refnum<class "Actor.lvclass">)  [unwired: 8 in]
  n119 = Unregister For Events(event registration refnum=w17) -> ()  [unwired: 1 in, 1 out]
  "String Indicator" <- "" ("String Indicator")
